vi "AuMT8852B Output Power Extended Results Query.vi"(7 "Stage":T1(ring), 8 "error in (no error)":errorcluster, 11 "VISA session":refnum<visa-resource-name>) -> (0 "error out":errorcluster, 2 "error code":i32, 3 "VISA session out":refnum<visa-resource-name>, 4 "Results":T2 {"Test peak power" format="%.2f"; "Test average power, min" format="%.2f"; "Test average power, max" format="%.2f"; "Packet average power" format="%.2f"})   [LabVIEW 2017]
doc: "Anritsu MT8852B Bluetooth Tester\n\nReturns the results of the Output Power test.\n\nINPUTS\nStage - results of the individual hopping stages of the test.\n\nOUTPUTS\nResults - measurements made during the test."
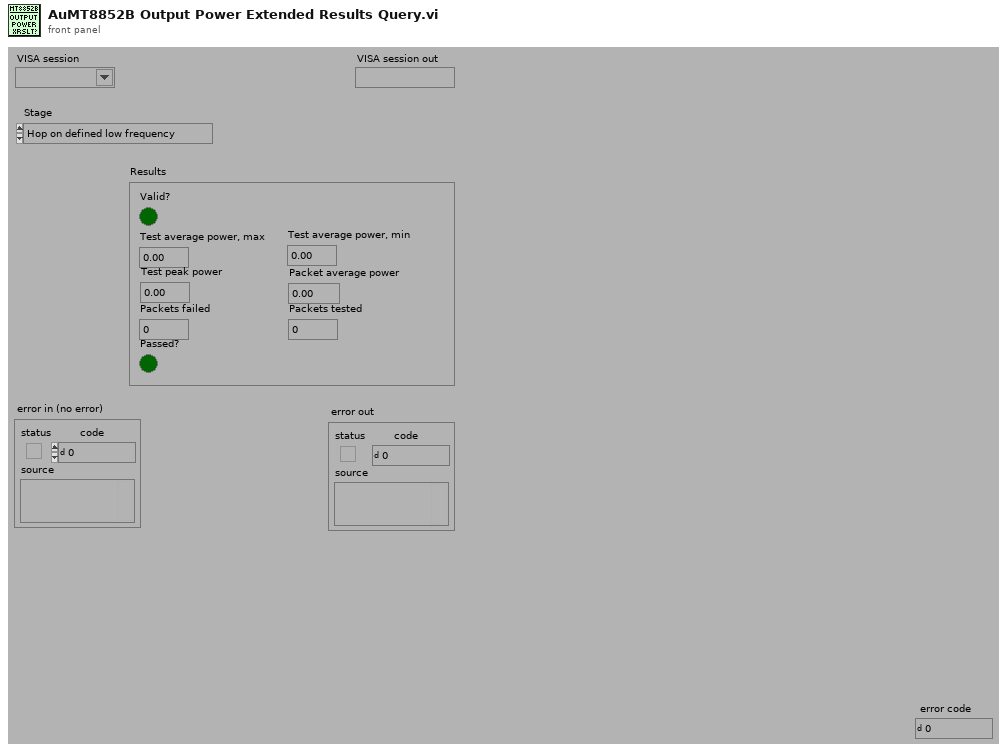
[diagram p1: front panel]
types:
  T1 = enum16{"Hop on defined low frequency", "Hop on defined medium frequency", "Hop on defined high frequency", "Hop on all channels", "Hop on any channels", "Hop off defined low frequency", "Hop off defined medium frequency", "Hop off defined high frequency"}
  T2 = cluster{"Valid?":bool, "Packet average power":dbl, "Test average power, max":dbl, "Test average power, min":dbl, "Test peak power":dbl, "Passed?":bool, "Packets failed":i32, "Packets tested":i32}
  T3 = enum16{"Simulate", "Range check", "Cache", "Query instrument status"}
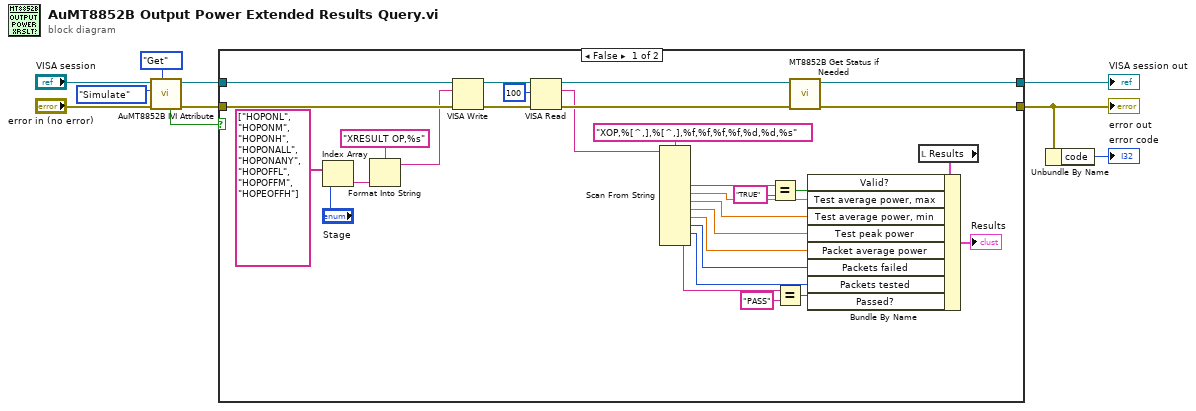
[diagram p0: block diagram]
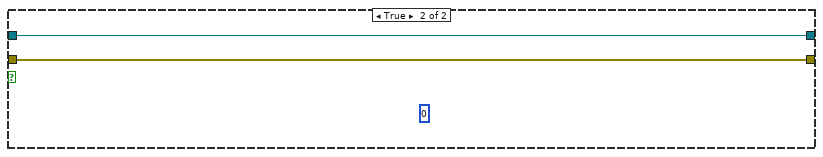
[diagram p2: hidden frame]
diagram:
  n1 = call <instrlib>:"AuMT8852B IVI Attribute.vi"("Set/Get (Set)"=enum16{"Set", "Get"}."Get", "error in (no error)"="error in (no error)", "Flag (Simulate)"=T3."Simulate", "VISA session"="VISA session") -> ("error out"=w7:errorcluster, "VISA session out"=w9:refnum<visa-resource-name>, "Value out"=w3:bool)  [unwired: 5 in]
  n2 = case shown="False" w3 {
    tunnel: [w30 w42] -> w10
    tunnel: [w29 w41] -> w1
    tunnel: w9 -> [w40 w42]
    tunnel: w7 -> [w39 w41]
    frame False {
      n3 = Index Array(array=string[] ["HOPONL", "HOPONM", "HOPONH", "HOPONALL", "HOPONANY", "HOPOFFL", "HOPOFFM", "HOPEOFFH"], index="Stage") -> (element=w23:string)
      n4 = Format Into String(format string="XRESULT OP,%s" ("write buffer (\"\")"), w23) -> (resulting string=w25:string)  [unwired: 2 in, 1 out]
      n5 = VISA Write(VISA resource name=w40, write buffer=w25, error in (no error)=w39) -> (VISA resource name out=w38:refnum<visa-resource-name>, error out=w37:errorcluster)  [unwired: 1 out]
      n6 = VISA Read(VISA resource name=w38, byte count=u32 100 ("byte count (0)"), error in (no error)=w37) -> (VISA resource name out=w28:refnum<visa-resource-name>, read buffer=w11:string, error out=w27:errorcluster)  [unwired: 1 out]
      n7 = Scan From String(format string="XOP,%[^,],%[^,],%f,%f,%f,%f,%d,%d,%s" ("Format String"), input string=w11) -> (output 2=w21:string, output 3=w20:dbl, output 4=w19:dbl, output 5=w18:dbl, output 6=w17:dbl, output 7=w13:i32, output 8=w12:i32, output 9=w14:string)  [unwired: 12 in, 3 out]
      n8 = Equal?(x=w21, y="TRUE") -> (x = y?=w33:bool)
      n9 = Equal?(x=w14, y="PASS") -> (x = y?=w16:bool)
      n10 = call <instrlib>:"MT8852B Get Status if Needed.vi"("error in (no error)"=w27, "VISA session"=w28) -> ("error out"=w29:errorcluster, "VISA session out"=w30:refnum<visa-resource-name>)  [unwired: 8 in]
      n11 = local read "Results"() -> (w34:T2)
      n12 = Bundle By Name(cluster=w34, "Valid?"=w33, "Test average power, max"=w20, "Test average power, min"=w19, "Test peak power"=w18, "Packet average power"=w17, "Packets failed"=w13, "Packets tested"=w12, "Passed?"=w16) -> (→"Results":T2)
    }
    frame True {
      (unwired) u8 0
    }
  }
  "error out" <- w1
  "VISA session out" <- w10
  n13 = Unbundle By Name(w1) -> ("code"=→"error code":i32)
